vi "Direction Status.vi"(10 "Direction":T2, 11 "Square":refnum<class "Square.lvclass">) -> (1 "Team Index":i32, 2 "Status":T1)   [LabVIEW 2020, in "SquareBattle.lvlib" / "Square.lvclass"]
doc: "Provides the status of a neighboring position specified by the direction from this square to check. The returned status cluster specifies whether the location is empty, contains a friend, or contains an enemy."
uses:
  Square.lvclass
  Direction.ctl
  Location Status.ctl
  Square.lvclass/Square.ctl
  SquareBattle.lvlib
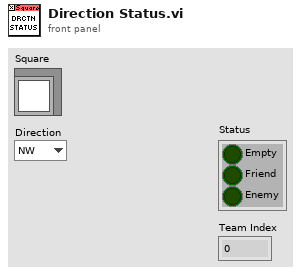
[diagram p1: front panel]
types:
  T1 = typedef "SquareBattle.lvlib/Location Status.ctl" = cluster{"Empty":bool, "Friend":bool, "Enemy":bool}
  T2 = typedef "SquareBattle.lvlib/Direction.ctl" = enum16{"NW", "N", "NE", "E", "SE", "S", "SW", "W"}
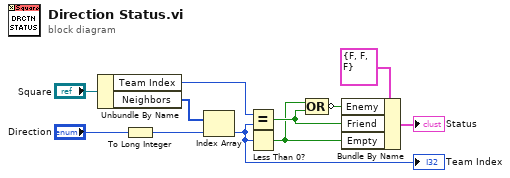
[diagram p0: block diagram]
diagram:
  n1 = Unbundle By Name("Square") -> ("Team Index"=w6:i32, "Neighbors"=w9:i32[])
  n2 = To Long Integer(number="Direction") -> (32bit integer=w2:i32)
  n3 = Index Array(array=w9, index=w2) -> (element=w1:i32)
  "Team Index" <- w1
  n4 = Equal?(x=w6, y=w1) -> (x = y?=w4:bool)
  n5 = Less Than 0?(x=w1) -> (x < 0?=w3:bool)
  n6 = Compound Arithmetic op=OR(w3, w4) -> (invert w5:bool)
  n7 = Bundle By Name(cluster=T1 {"Empty"=FALSE, "Friend"=FALSE, "Enemy"=FALSE} ("Status"), "Enemy"=w5, "Friend"=w4, "Empty"=w3) -> (→"Status":T1)
